vi "Memory write from DMA - Target.vi"   [LabVIEW 2014]
uses:
  <vilib>/Platform/TimedLoop/XDataNode/timing_clust.ctl
  <vilib>/Platform/TimedLoop/XDataNode/nitl_modes.ctl
  <vilib>/Platform/TimedLoop/XDataNode/wakeup.ctl
  <vilib>/rvi/Emulation/niFpgaSctlEmulationGetInTimedLoop.vi
  <vilib>/rvi/Emulation/niFpgaEmulationReportErrorSimple.vi
  <vilib>/rvi/Emulation/niFpgaGetClockAttributes.vi
  <vilib>/rvi/Emulation/niFpgaCriticalErrorInLSC.vi
  <vilib>/rvi/interface/RandomDataEmulation/niFpgaRandomDataHandleErrors.vi
  <vilib>/rvi/Memory/Memory_Emulation/nirvimemoryFastEmulation.vi
  <vilib>/rvi/Memory/Memory_Emulation/nirvimemoryEmulation.vi
  <vilib>/rvi/Emulation/niFpgaEmulationIsFPGAContextNoSignature.vi
  <vilib>/rvi/DataTransferAndStorage/Container/Common/niFpgaContainerGetUniqueNameForEmu.vi
  <vilib>/rvi/Emulation/niFpgaProcessEmulError.vi
  <vilib>/rvi/errors/nirviReportUnexpectedCaseInternalError (U32).vi
  <vilib>/Platform/TimedLoop/XDataNode/XDataNode.xnode
  <vilib>/rvi/DataTransferAndStorage/Container/XNode/niFpgaContainer.xnode
  <vilib>/rvi/interface/RandomDataEmulation/nirviRandomDataFpgaReadWriteTemplate.vi
  <vilib>/Platform/TimedLoop/XDataNode/XDNodeRunTimeDep.lvlib
types:
  T1 = typedef "XDNodeRunTimeDep.lvlib/timing_clust.ctl" = cluster{"Expected End [f-1]":u64, "Actual End [f-1]":u64, "Finished Late? [f-1]":bool, "Expected End [i-1]":u64, "Actual End [i-1]":u64, "Finished Late? [i-1]":bool, "Expected Start [i]":u64, "Actual Start [i]":u64, "Expected Start [f]":u64, "Actual Start [f]":u64, "Source Name":string, "Structure Name":string, "Period":i64, "Deadline":i64, "Offset":i64, "Start":i64, "Priority":i32, "Timeout":i32, "Mode":T2, "Wakeup Reason":T3, "Error":errorcluster, "Source Type":string, "Secondary Source Type":string, "Global End Time":u64, "Global Start Time":u64, "Frame Duration":u64, "Iteration Duration":u64, "Assigned CPU":i32, "I/O Scan Engine Mode":u32}
  T2 = typedef "XDNodeRunTimeDep.lvlib/nitl_modes.ctl" = enum32{"No Change", "Process missed periods, maintain original phase", "Discard missed periods, maintain original phase", "Process missed periods, ignore original phase", "Discard missed periods, ignore original phase"}
  T3 = typedef "XDNodeRunTimeDep.lvlib/wakeup.ctl" = enum32{"Normal", "Aborted", "Asynchronous wakeup", "Timing source error", "Timed loop error", "Timeout"}
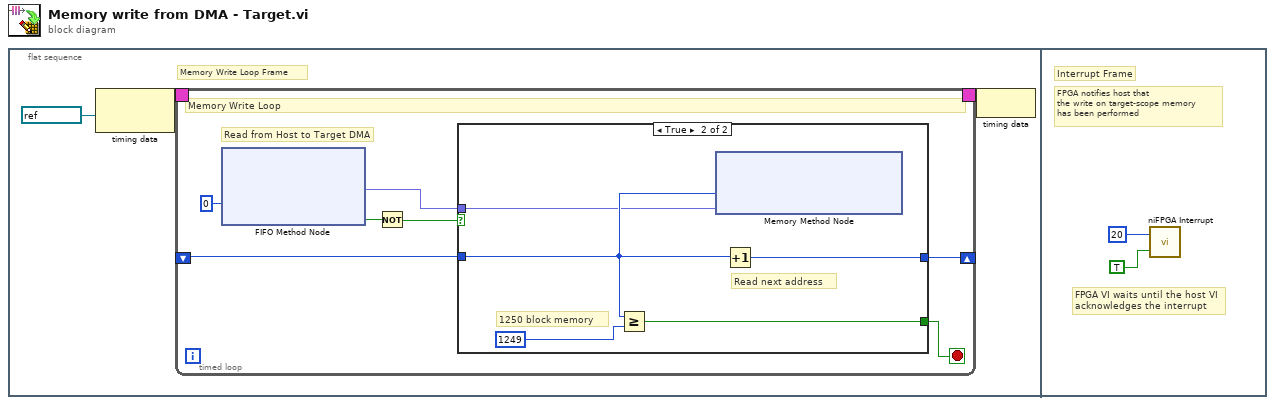
[diagram p0: block diagram]
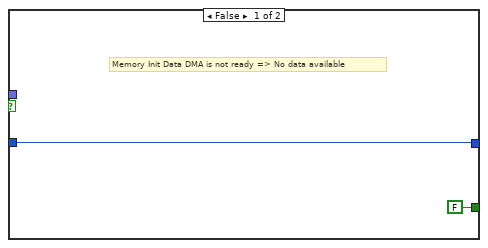
[diagram p2: hidden frame]
diagram:
  n1 = flat-sequence {
    frame #0 {
      # "Memory Write Loop Frame"
      n2 = node-c288(refnum<k21> "50MHz" ("Source Name")) -> (w3:T1)
      n3 = timed-loop {
        shift-right: [w8] -> _
        shift-left: _ -> [w9]
        timing: w3 -> [_]
        timing-out: [_] -> w2
        stop <- w10 stop-if-true
        # "Read from Host to Target DMA"
        # "Memory Write Loop"
        n4 = xnode ("FIFO Method Node")("Timeout"=0) -> ("Element"=w4:fxp<+/-,12,12>, "Timed Out?"=w6:bool)  [unwired: 1 in, 1 out]
        n5 = Not(x=w6) -> (.not. x?=w5:bool)
        n6 = case shown="True" w5 {
          tunnel: [FALSE w16] -> w10
          tunnel: w9 -> [w11 w15]
          tunnel: [w11 w14] -> w8
          tunnel: w4 -> [_ w13]
          frame False {
            # "Memory Init Data DMA is not ready => No data available"
          }
          frame True {
            # "Read next address"
            # "1250 block memory"
            n7 = Greater Or Equal?(x=w15, y=u32 1249) -> (x >= y?=w16:bool)
            n8 = xnode ("Memory Method Node")("Address"=w15, "Data"=w13) -> ()  [unwired: 1 in, 1 out]
            n9 = Increment(x=w15) -> (x+1=w14:u32)
          }
        }
      }
      n10 = node-c288(w2) -> ()
    }
    frame #1 {
      # "FPGA VI waits until the host VI \nacknowledges the interrupt"
      # "FPGA notifies host that\nthe write on target-scope memory\nhas been performed"
      # "Interrupt Frame"
      n11 = call <vilib>:"niFPGA Interrupt.vi"("Wait Until Cleared (F)"=TRUE, "IRQ Number (0)"=u8 20) -> ()  [unwired: 1 in]
    }
  }
